vi "control a led by a switch (arduino).vi"() -> ()   [LabVIEW 2019]
uses:
  <vilib>/LabVIEW Interface for Arduino/Type Defs/Board Type.ctl
  <vilib>/LabVIEW Interface for Arduino/Type Defs/Connection Type.ctl
  <vilib>/LabVIEW Interface for Arduino/Type Defs/Pin Mode.ctl
  <vilib>/LabVIEW Interface for Arduino/LabVIEW Interface for Arduino.lvlib
panel:
  in  "Boolean":bool
  in  "Digital I/O Pin (0)":u8
  in  "Digital I/O Pin":u8
  in  "Bytes Per Packet (15)":u32=15
  in  "VISA resource":refnum<visa-resource-name>
  in  "stop":bool
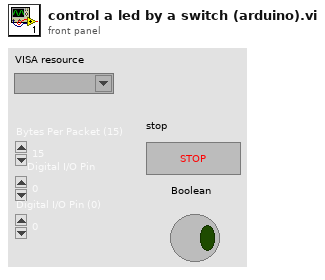
[diagram p1: front panel]
types:
  T1 = typedef "LabVIEW Interface for Arduino.lvlib/Pin Mode.ctl" = enum8{"Input", "Output"}
  T2 = typedef "LabVIEW Interface for Arduino.lvlib/Connection Type.ctl" = enum8{"USB / Serial", "XBEE", "BlueSmirf (Bluetooth)"}
  T3 = typedef "LabVIEW Interface for Arduino.lvlib/Board Type.ctl" = enum16{"Uno", "Dimuelanove w/Atmega 328", "Mega 2560"}
  T4 = typedef "LabVIEW Interface for Arduino.lvlib/Arduino Resource.ctl" = cluster{"VISA resource":refnum<visa-resource-name>, "Board Type":T3, "Connection Type":enum8{"USB / Serial"}, "Bytes Per Packet (15)":u8}
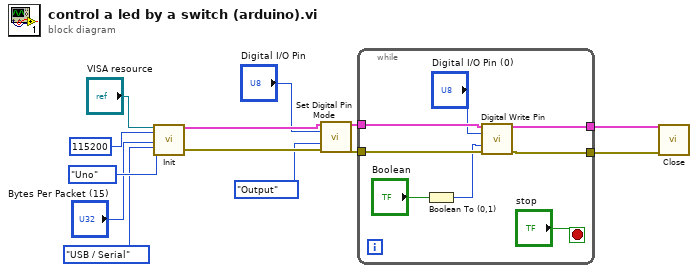
[diagram p0: block diagram]
diagram:
  n1 = call <vilib>:"Init.vi"("VISA resource"="VISA resource", "Baud Rate (115200)"=u32 115200, "Board Type (Uno)"=Board_Type."Uno", "Bytes Per Packet (15)"="Bytes Per Packet (15)", "Connection Type (USB/Serial)"=Connection_Type."USB / Serial") -> ("Arduino Resource"=w8:T4, "error out"=w9:errorcluster)  [unwired: 13 in]
  n2 = call <vilib>:"Set Digital Pin Mode.vi"("Arduino Resource"=w8, "Digital I/O Pin"="Digital I/O Pin", "Pin Mode (Input)"=Pin_Mode."Output", "error in"=w9) -> ("Arduino Resource"=w13:T4, "error out"=w10:errorcluster)  [unwired: 10 in]
  n3 = while {
    tunnel: w13 -> [w20]
    tunnel: [w19] -> w12
    tunnel: [w18] -> w11
    tunnel: w10 -> [w17]
    stop <- "stop" stop-if-true
    n4 = Boolean To (0,1)(Boolean="Boolean") -> (0, 1=w14:i16)
    n5 = call <vilib>:"Digital Write Pin.vi"("Arduino Resource"=w20, "Digital I/O Pin (0)"="Digital I/O Pin (0)", "Value (0)"=w14, "error in"=w17) -> ("Arduino Resource"=w19:T4, "error out"=w18:errorcluster)  [unwired: 10 in]
  }
  n6 = call <vilib>:"Close.vi"("Arduino Resource"=w12, "error in"=w11) -> ()  [unwired: 13 in, 1 out]
